vi "getStageFromXml.vi"(8 "error in (no error)":errorcluster, 10 "Xml":refnum<class "xmlNode.lvclass">, 11 "ScriptEvent in":refnum<class "ScriptEvent.lvclass">) -> (0 "error out":errorcluster, 2 "Xml out":refnum<class "xmlNode.lvclass">, 3 "ScriptEvent out":refnum<class "ScriptEvent.lvclass">)   [LabVIEW 2009, in "Tools.lvlib" / "Scripting.lvlib" / "ScriptEvent.lvclass"]
uses:
  ScriptEvent.lvclass
  xmlNode/xmlNode.lvclass
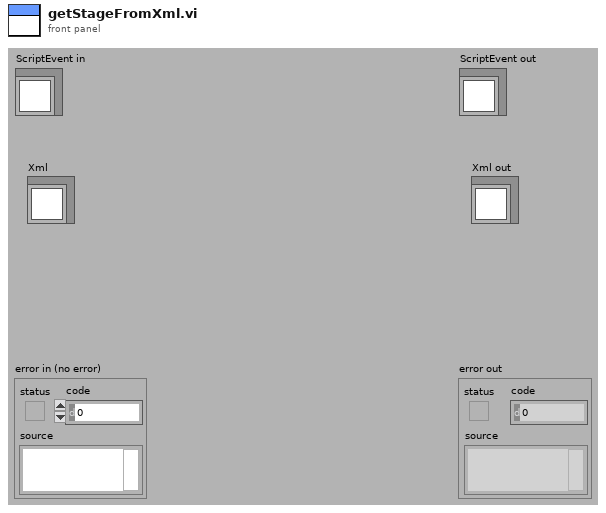
[diagram p1: front panel]
types:
  T1 = enum16{"Initialise", "MOT", "Molasses", "Optical Pumping", "Magnetic Trap", "RF Cooling", "Manipulation", "Switch Off", "Absorption Imaging", "Fluorscence Imaging", "Shut Down"}
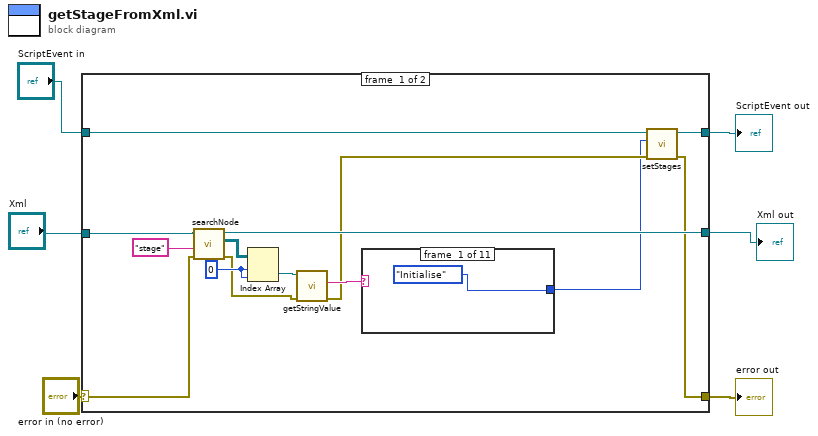
[diagram p0: block diagram]
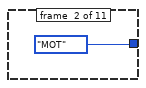
[diagram p2: hidden frame]
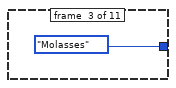
[diagram p3: hidden frame]
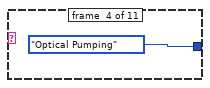
[diagram p4: hidden frame]
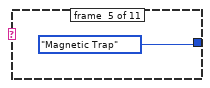
[diagram p5: hidden frame]
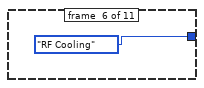
[diagram p6: hidden frame]
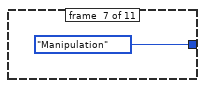
[diagram p7: hidden frame]
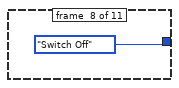
[diagram p8: hidden frame]
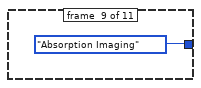
[diagram p9: hidden frame]
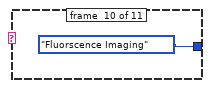
[diagram p10: hidden frame]
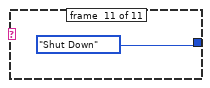
[diagram p11: hidden frame]
diagram:
  n1 = case shown="No Error" "error in (no error)" {
    selector: "error in (no error)" -> [w14 w33]
    tunnel: [w7 w33] -> w5
    tunnel: [w11 w32] -> w3
    tunnel: "ScriptEvent in" -> [w10 w32]
    tunnel: "Xml" -> [w16 _]
    tunnel: [w15 _] -> w1
    frame #0 {
      w18 = 0
      n2 = call-dynamic "searchNode.vi"("error in (no error)"=w14, "searchElementName"="stage", "xmlNode in"=w16) -> ("error out"=w13:errorcluster, "arrayXmlNodes"=w19:refnum<class "xmlNode.lvclass">[][], "xmlNode out"=w15:refnum<class "xmlNode.lvclass">)  [unwired: 6 in]
      n3 = Index Array(array=w19, index (row)=w18, index (col)=w18) -> (element=w17:refnum<class "xmlNode.lvclass">)
      n4 = call-dynamic "getStringValue.vi"("error in (no error)"=w13, "xmlNode.lvclass in"=w17) -> ("error out"=w9:errorcluster, "stringValue"=w12:string)  [unwired: 7 in, 1 out]
      n5 = case shown="\"Manipulation\"" w12 {
        tunnel: [T1."Initialise" ("Value") T1."MOT" ("Value") T1."Molasses" ("Value") T1."Optical Pumping" ("Value") T1."Magnetic Trap" ("Value") T1."RF Cooling" ("Value") T1."Manipulation" ("Value") T1."Switch Off" ("Value") T1."Absorption Imaging" ("Value") T1."Fluorscence Imaging" ("Value") T1."Shut Down" ("Value")] -> w8
        frame #0 {
        }
        frame #1 {
        }
        frame #2 {
        }
        frame #3 {
        }
        frame #4 {
        }
        frame #5 {
        }
        frame #6 {
        }
        frame #7 {
        }
        frame #8 {
        }
        frame #9 {
        }
        frame #10 {
        }
      }
      n6 = call-dynamic "setStages.vi"("error in (no error)"=w9, "Stage"=w8, "ScriptEvent.lvclass in"=w10) -> ("error out"=w7:errorcluster, "ScriptEvent.lvclass out"=w11:refnum<class "ScriptEvent.lvclass">)  [unwired: 7 in]
    }
    frame #1 {
    }
  }
  "error out" <- w5
  "ScriptEvent out" <- w3
  "Xml out" <- w1
